vi "local barometric pressure.vi"() -> (1 "Atmospheric pressure":dbl[unit], 2 "Atmospheric pressure (kPa)":dbl)   [LabVIEW 2015]
panel:
  out "data":string
  out "error out":errorcluster
  in  "http URL":string="www.cornell.edu/weather/"
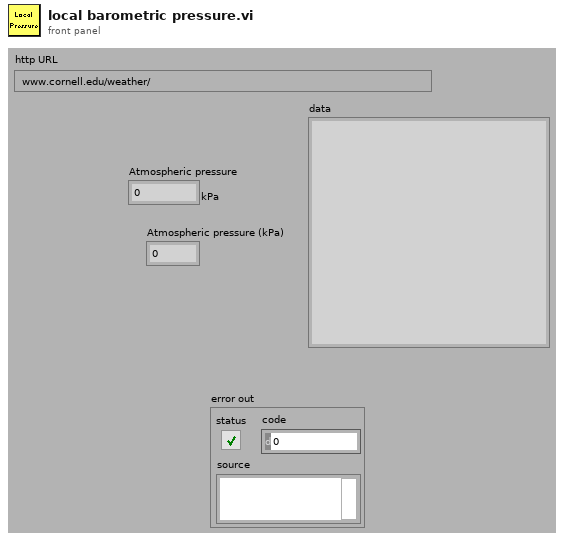
[diagram p1: front panel]
types:
  T1 = enum16{"Read", "Write", "ReadWrite", "BufferedRead", "BufferedReadWrite"}
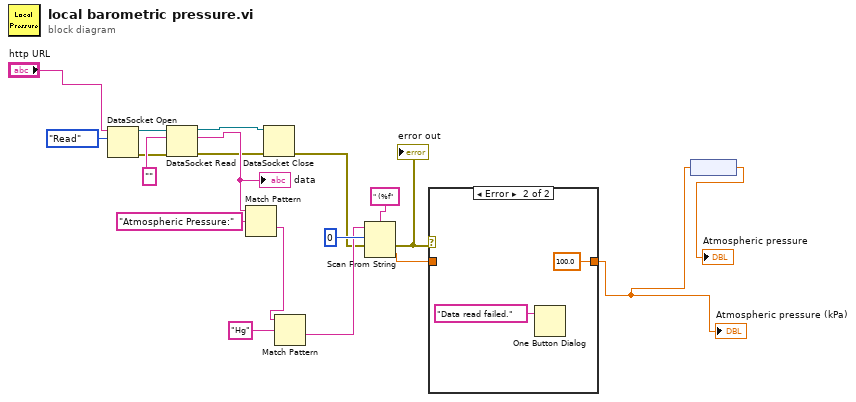
[diagram p0: block diagram]
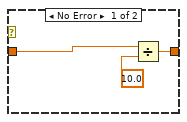
[diagram p2: hidden frame]
diagram:
  n1 = DataSocket Open(10:T1."Read" ("mode"), 11:"http URL") -> (0:w5:errorcluster, 3:w4:refnum<k13>)  [unwired: 2 in]
  n2 = DataSocket Read(8:w5, 10:"" ("http URL"), 11:w4) -> (0:w2:errorcluster, 2:w14:string, 3:w3:refnum<k13>)  [unwired: 2 in, 4 out]
  "data" <- w14
  n3 = Match Pattern(string=w14, regular expression="Atmospheric Pressure:") -> (after substring=w12:string)  [unwired: 1 in, 3 out]
  n4 = DataSocket Close(8:w2, 11:w3) -> (0:w1:errorcluster)  [unwired: 1 in, 1 out]
  n5 = Match Pattern(string=w12, regular expression="Hg") -> (after substring=w10:string)  [unwired: 1 in, 3 out]
  n6 = Scan From String(format string=" (%f", input string=w10, initial scan location=u32 0, error in=w1) -> (error out=w13:errorcluster, output 1=w16:dbl)  [unwired: 1 in, 2 out]
  "error out" <- w13
  n7 = case shown="Error" w13 {
    tunnel: w16 -> [w22 _]
    tunnel: [w20 100.0] -> w9
    frame No Error {
      n8 = Divide(x=w22, y=10.0) -> (x/y=w20:dbl)
    }
    frame Error {
      n9 = One Button Dialog(message="Data read failed.") -> ()  [unwired: 1 in, 1 out]
    }
  }
  "Atmospheric pressure (kPa)" <- w9
  n10 = node(w9) -> (→"Atmospheric pressure":dbl[unit])
